vi "libssh2_channel_request_pty.vi"(8 "error in (no error)":errorcluster, 10 "term":string, 11 "channel":T1) -> (0 "error out":errorcluster)   [LabVIEW 2017, in "libssh2.lvlib"]
doc: "Request a pseudo-terminal with a default width of 80 columns and 24 rows on a channel."
uses:
  libssh2.lvlib
  Channel Refnum.ctl
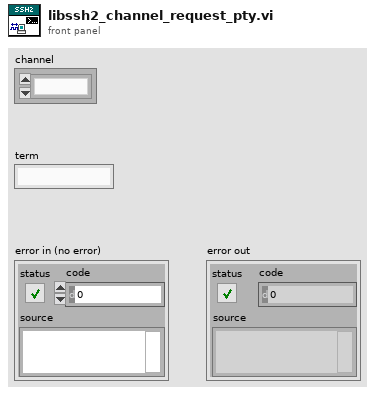
[diagram p1: front panel]
types:
  T1 = typedef "libssh2.lvlib/Channel Refnum.ctl" = refnum<k1>
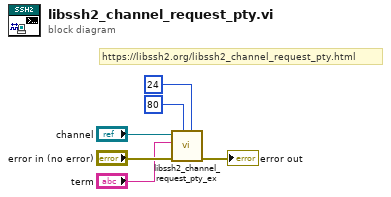
[diagram p0: block diagram]
diagram:
  # "https://libssh2.org/libssh2_channel_request_pty.html"
  n1 = call "libssh2_channel_request_pty_ex.vi"("height"=24, "width"=80, "error in (no error)"="error in (no error)", "term"="term", "channel"="channel") -> ("error out"=→"error out":errorcluster)  [unwired: 6 in]
